vi "Start Chef Initialization.vi"(8 "error in (no error)":errorcluster, 11 "Chef Actor in":refnum<class "Chef Actor.lvclass">) -> (0 "error out":errorcluster, 3 "Chef Actor out":refnum<class "Chef Actor.lvclass">)   [LabVIEW 2024, in "Chef Actor.lvlib" / "Chef Actor.lvclass"]
uses:
  Chef Actor.lvclass
  Chef Actor.lvclass/Chef Actor.ctl
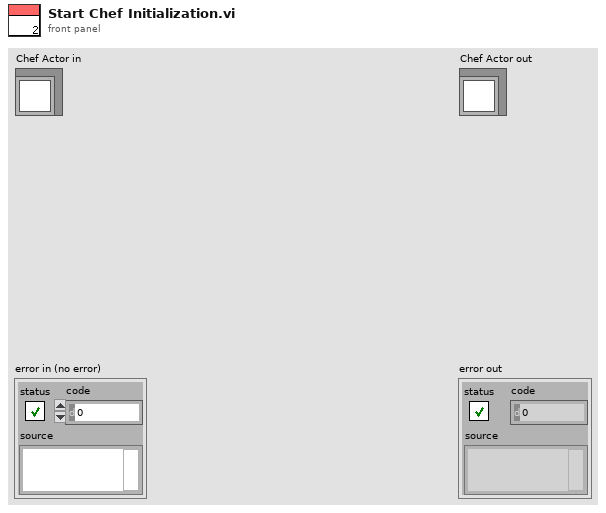
[diagram p1: front panel]
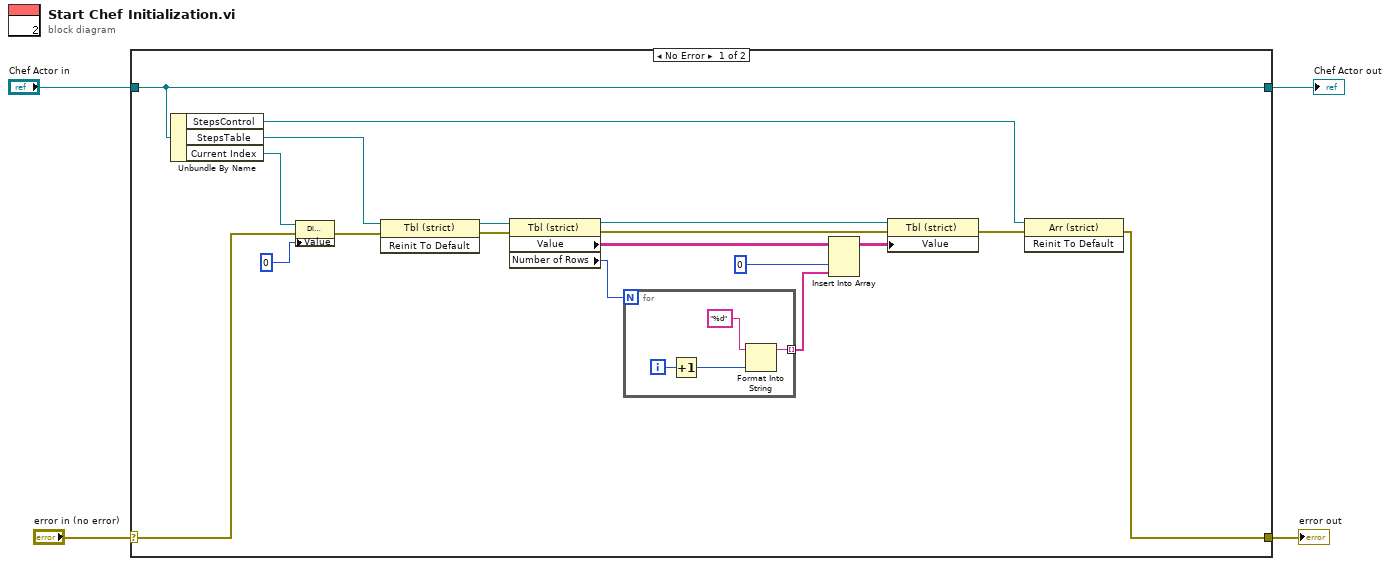
[diagram p0: block diagram]
diagram:
  n1 = case shown="No Error" "error in (no error)" {
    selector: "error in (no error)" -> [w5 w28]
    tunnel: [w9 w28] -> w3
    tunnel: [w22 w27] -> w1
    tunnel: "Chef Actor in" -> [w22 w27]
    frame No Error {
      n2 = Unbundle By Name(w22) -> ("StepsControl"=w11:refnum<vi>, "StepsTable"=w21:refnum<vi>, "Current Index"=w8:refnum<vi>)
      n3 = property class="DigNum (strict)"(reference=w8, error in=w5, "Value"=0) -> (error out=w7:errorcluster)  [unwired: 1 out]
      n4 = invoke class="Tbl (strict)" method="Reinit To Default"(reference=w21, error in=w7) -> (reference out=w20:refnum<vi>, error out=w19:errorcluster)  [unwired: 1 in, 1 out]
      n5 = property class="Tbl (strict)"(reference=w20, error in=w19) -> (reference out=w12:refnum<vi>, error out=w13:errorcluster, "Value"=w17:string[][], "Number of Rows"=w18:u32)
      n6 = for {
        N: w18 -> [_]
        tunnel: [w24] -> w16 mode=indexing
        i -> [w26]
        n7 = Increment(x=w26) -> (x+1=w23:i32)
        n8 = Format Into String(format string="%d", w23) -> (resulting string=w24:string)  [unwired: 2 in, 1 out]
      }
      n9 = Insert Into Array(array=w17, index (col)=0, new element=w16) -> (w14:string[][])  [unwired: 1 in]
      n10 = property class="Tbl (strict)"(reference=w12, error in=w13, "Value"=w14) -> (error out=w10:errorcluster)  [unwired: 1 out]
      n11 = invoke class="Arr (strict)" method="Reinit To Default"(reference=w11, error in=w10) -> (error out=w9:errorcluster)  [unwired: 1 in, 2 out]
    }
    frame Error {
    }
  }
  "error out" <- w3
  "Chef Actor out" <- w1
